vi "load.vi"(8 "error in (no error)":errorcluster caption="entrée d'erreur (pas d'erreur)", 11 "Model.lvclass":refnum<class "Model.lvclass">) -> (0 "error out":errorcluster caption="sortie d'erreur", 2 "loaded_model":string, 3 "Model.lvclass 2":refnum<class "Model.lvclass">)   [LabVIEW 2020, in "Model.lvclass"]
doc: "Load a trained model."
uses:
  Model.lvclass
  C:/Users/cipop/TDF Dropbox/2_Technologies de France/1 - Services et Etudes/PLAIY/2 - DEV/PLAIYLAB/code/Python/Python.lvclass
  Model.lvclass/Model.ctl
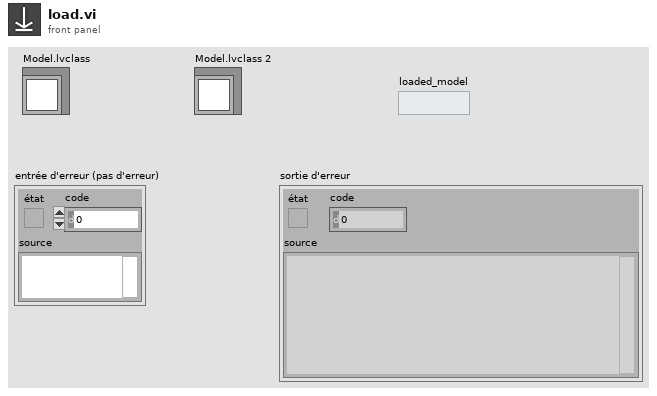
[diagram p1: front panel]
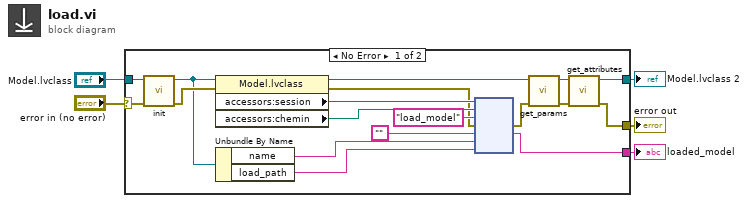
[diagram p0: block diagram]
diagram:
  n1 = case shown="No Error" "error in (no error)" {
    selector: "error in (no error)" -> [w16 w25]
    tunnel: [w10 w25] -> w4
    tunnel: [w9 w24] -> w2
    tunnel: "Model.lvclass" -> [w17 w24]
    tunnel: [w19 _] -> w1
    frame No Error {
      n2 = call-dynamic "init.vi"("error in (no error)"=w16, "Model en entrée"=w17) -> ("error out"=w15:errorcluster, "Model en sortie"=w8:refnum<class "Model.lvclass">)  [unwired: 8 in]
      n3 = property class="Model.lvclass"(reference=w8, error in=w15) -> (reference out=w14:refnum<class "Model.lvclass">, error out=w18:errorcluster, "accessors:session"=w22:refnum<k35>, "accessors:chemin"=w21:path)
      n4 = Unbundle By Name(w8) -> ("name"=w7:string, "load_path"=w6:string)
      n5 = node(w22, w21, "load_model" ("nom de la fonction"), w18, "", w7, w6) -> (w13:errorcluster, w19:string)  [unwired: 2 in, 3 out]
      n6 = call-dynamic "get_params.vi"("error in (no error)"=w13, "Model en entrée"=w14) -> ("error out"=w11:errorcluster, "Model en sortie"=w12:refnum<class "Model.lvclass">)  [unwired: 8 in]
      n7 = call-dynamic "get_attributes.vi"("error in (no error)"=w11, "Model en entrée"=w12) -> ("error out"=w10:errorcluster, "Model en sortie"=w9:refnum<class "Model.lvclass">)  [unwired: 8 in]
    }
    frame Error {
    }
  }
  "error out" <- w4
  "Model.lvclass 2" <- w2
  "loaded_model" <- w1
